vi "DIVISION.vi"(9 "r":dbl[](array[numeric]), 10 "dr":dbl[](array[numeric])) -> (2 "dr/r":dbl[](array[numeric]))   [LabVIEW 2016]
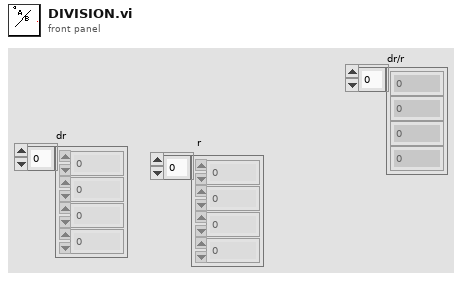
[diagram p1: front panel]
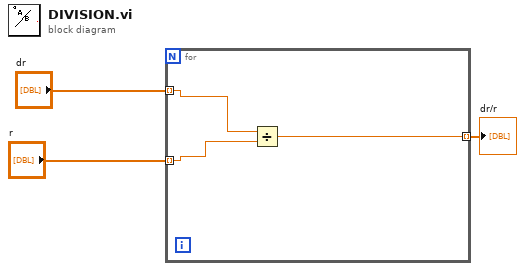
[diagram p0: block diagram]
diagram:
  n1 = for {
    tunnel: "dr" -> [w6] mode=indexing
    tunnel: "r" -> [w5] mode=indexing
    tunnel: [w4] -> w1 mode=indexing
    n2 = Divide(x=w6, y=w5) -> (x/y=w4:dbl)
  }
  "dr/r" <- w1
